vi "TCP read variable.vi"(0 "connection ID":refnum<k5>, 9 "timeout ms (25000)":i32=25000, 11 "error in (no error)":errorcluster) -> (4 "connection ID out":refnum<k5>, 6 "bytes read":i32, 8 "data out":string, 15 "error out":errorcluster)   [LabVIEW 2015]
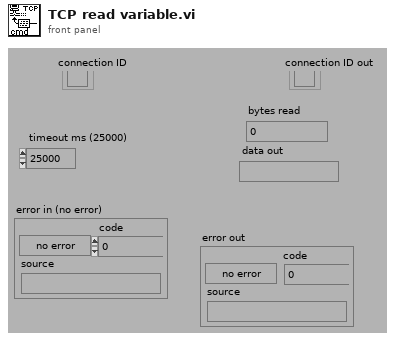
[diagram p1: front panel]
types:
  T1 = enum16{"Standard", "Buffered", "CRLF", "Immediate"}
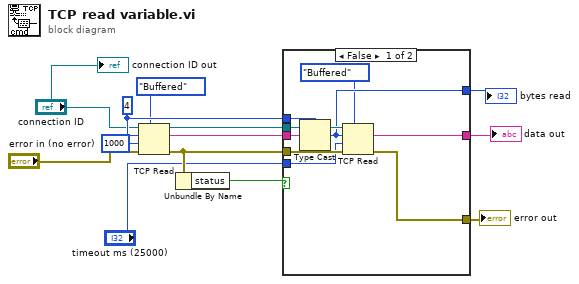
[diagram p0: block diagram]
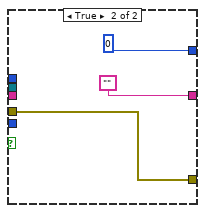
[diagram p2: hidden frame]
diagram:
  w13 = 4
  n1 = TCP Read(connection ID="connection ID", bytes to read=w13, error in (no error)="error in (no error)", 7:T1."Buffered" ("mode (standard)"), 9:1000 ("timeout ms (25000)")) -> (connection ID out=w11:refnum<k5>, data out=w12:string, error out=w8:errorcluster)
  n2 = Unbundle By Name(w8) -> ("status"=w7:bool)
  n3 = case shown="False" w7 {
    tunnel: w8 -> [w22 w25]
    tunnel: "timeout ms (25000)" -> [w21 _]
    tunnel: w11 -> [w20 _]
    tunnel: w12 -> [w19 _]
    tunnel: w13 -> [w18 _]
    tunnel: [w17 w25] -> w6
    tunnel: [w16 ""] -> w5
    tunnel: [w15 0] -> w4
    frame False {
      n4 = Type Cast(type=w18, x=w19) -> (*(type *) &x=w15:i32)
      n5 = TCP Read(connection ID=w20, bytes to read=w15, error in (no error)=w22, 7:T1."Buffered" ("mode (standard)"), 9:w21) -> (data out=w16:string, error out=w17:errorcluster)  [unwired: 1 out]
    }
    frame True {
    }
  }
  "error out" <- w6
  "data out" <- w5
  "bytes read" <- w4
  "connection ID out" <- "connection ID"
